vi "Magazine Control 4.0.vi"() -> ()   [LabVIEW 2020]
uses:
  2020 Infinite Recharge/2020 Infinite Recharge Styx Beta/Magazine State.ctl
  Documents/GitHub/TitanLib/Lib/TitanLib.lvlib
panel:
  in  "Magazine Overflow Power":dbl=1.0
  in  "Magazine Power":dbl=1.0
  in  "Intake Power":dbl=1.0
  out "Magazine":dbl
  out "Intake":dbl
  out "Current State":T1
  in  "Initial State":T1
  in  "Outtake Button":bool
  in  "Intake Button":bool
  in  "Exit Sensor":bool
  in  "Start Sensor":bool
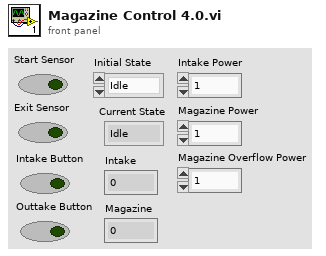
[diagram p1: front panel]
types:
  T1 = typedef "Magazine State.ctl" = enum16{"Idle", "Intake", "Index", "Prevent Overflow", "Outtake Idle", "Outtake"}
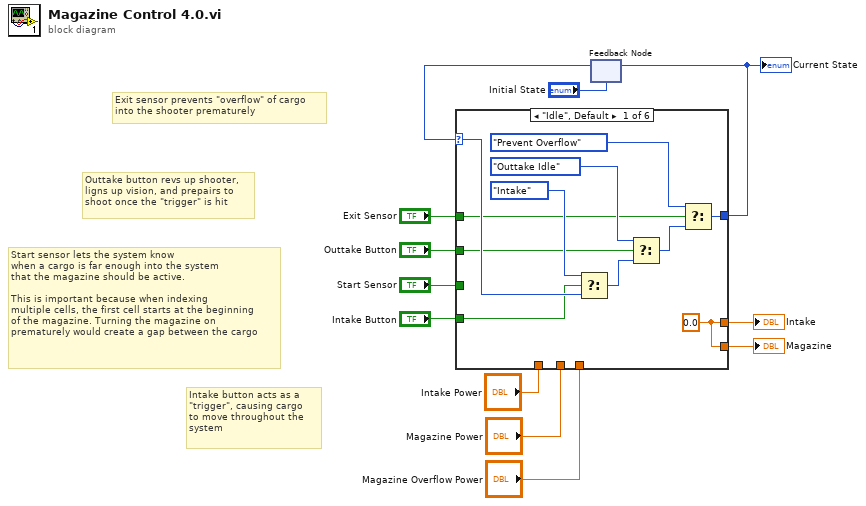
[diagram p0: block diagram]
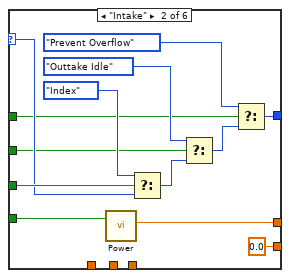
[diagram p2: hidden frame]
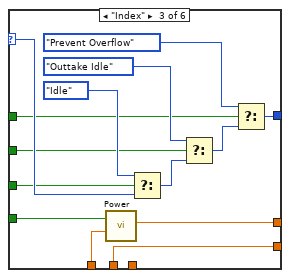
[diagram p3: hidden frame]
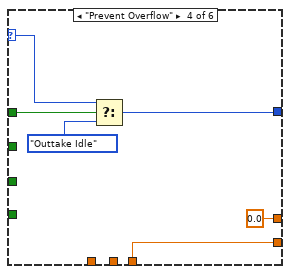
[diagram p4: hidden frame]
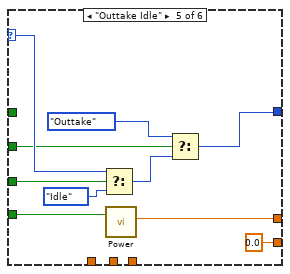
[diagram p5: hidden frame]
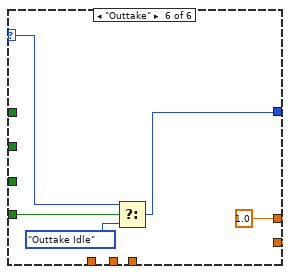
[diagram p6: hidden frame]
diagram:
  # "Start sensor lets the system know\nwhen a cargo is far enough into the system\nthat the magazine should be active.\n\nThis is important because when indexing\nmultiple cells, the first cell starts at the beginning\nof the magazine. Turning the magazine on\nprematurely would create a gap between the cargo"
  # "Exit sensor prevents \"overflow\" of cargo\ninto the shooter prematurely"
  # "Outtake button revs up shooter,\nligns up vision, and prepairs to\nshoot once the \"trigger\" is hit"
  # "Intake button acts as a\n\"trigger\", causing cargo\nto move throughout the \nsystem"
  n1 = feedback #1("Initial State") -> (w2:T1)
  n2 = case shown="\"Idle\", Default" w2 {
    selector: w2 -> [w17 w27 w41 w52 w62 w70]
    tunnel: "Intake Button" -> [w14 w34 w50 _ w66 w71]
    tunnel: [w23 w36 w49 0.0 ("Output") w65 w68] -> w10
    tunnel: [w23 0.0 w48 w56 0.0 ("Magazine Overflow Power") w68] -> w9
    tunnel: "Intake Power" -> [_ _ w47 _ _ _]
    tunnel: "Start Sensor" -> [_ w28 w38 _ w63 _]
    tunnel: "Magazine Power" -> [_ _ w48 _ _ _]
    tunnel: "Magazine Overflow Power" -> [_ _ _ w56 _ _]
    tunnel: "Outtake Button" -> [w15 w25 w39 _ w59 _]
    tunnel: "Exit Sensor" -> [w16 w26 w40 w53 _ _]
    tunnel: [w13 w24 w37 w51 w57 w67] -> w1
    frame "Idle", Default {
      w23 = 0.0
      n3 = Select(t=Magazine_State."Intake", s=w14, f=w17) -> (s? t:f=w18:T1)
      n4 = Select(t=Magazine_State."Outtake Idle" ("lower limit"), s=w15, f=w18) -> (s? t:f=w19:T1)
      n5 = Select(t=Magazine_State."Prevent Overflow" ("lower limit"), s=w16, f=w19) -> (s? t:f=w13:T1)
    }
    frame "Intake" {
      n6 = call "Power.vi"("Positive"=w34) -> ("Output"=w36:dbl)  [unwired: 10 in]
      n7 = Select(t=Magazine_State."Index", s=w28, f=w27) -> (s? t:f=w29:T1)
      n8 = Select(t=Magazine_State."Outtake Idle" ("lower limit"), s=w25, f=w29) -> (s? t:f=w30:T1)
      n9 = Select(t=Magazine_State."Prevent Overflow" ("lower limit"), s=w26, f=w30) -> (s? t:f=w24:T1)
    }
    frame "Index" {
      n10 = call "Power.vi"("Positive Power"=w47, "Positive"=w50) -> ("Output"=w49:dbl)  [unwired: 9 in]
      n11 = Select(t=Magazine_State."Idle", s=w38, f=w41) -> (s? t:f=w42:T1)
      n12 = Select(t=Magazine_State."Outtake Idle" ("lower limit"), s=w39, f=w42) -> (s? t:f=w43:T1)
      n13 = Select(t=Magazine_State."Prevent Overflow" ("lower limit"), s=w40, f=w43) -> (s? t:f=w37:T1)
    }
    frame "Prevent Overflow" {
      n14 = Select(t=w52, s=w53, f=Magazine_State."Outtake Idle" ("lower limit")) -> (s? t:f=w51:T1)
    }
    frame "Outtake Idle" {
      n15 = Select(t=w62, s=w63, f=Magazine_State."Idle") -> (s? t:f=w60:T1)
      n16 = call "Power.vi"("Positive"=w66) -> ("Output"=w65:dbl)  [unwired: 10 in]
      n17 = Select(t=Magazine_State."Outtake" ("f"), s=w59, f=w60) -> (s? t:f=w57:T1)
    }
    frame "Outtake" {
      w68 = 1.0 ("Magazine Overflow Power")
      n18 = Select(t=w70, s=w71, f=Magazine_State."Outtake Idle") -> (s? t:f=w67:T1)
    }
  }
  "Current State" <- w1
  "Intake" <- w10
  "Magazine" <- w9
  n19 = feedback-in #1(w1) -> ()
